vi "Read Voltage.vi"(8 "error in (no error)":errorcluster, 11 "Generic DAQ in":refnum<class "Generic DAQ.lvclass">) -> (0 "error out":errorcluster, 2 "Voltage":dbl, 3 "Generic DAQ out":refnum<class "Generic DAQ.lvclass">)   [LabVIEW 2020, in "Generic DAQ.lvclass"]
uses:
  Generic DAQ.lvclass
  <vilib>/numeric/Random Number (Range) DBL.vi
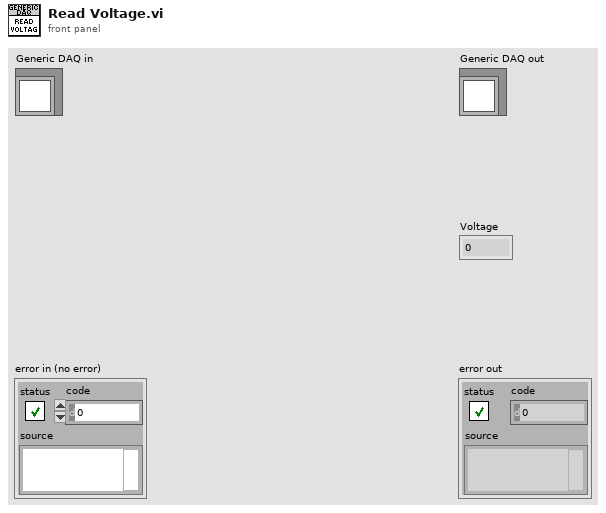
[diagram p1: front panel]
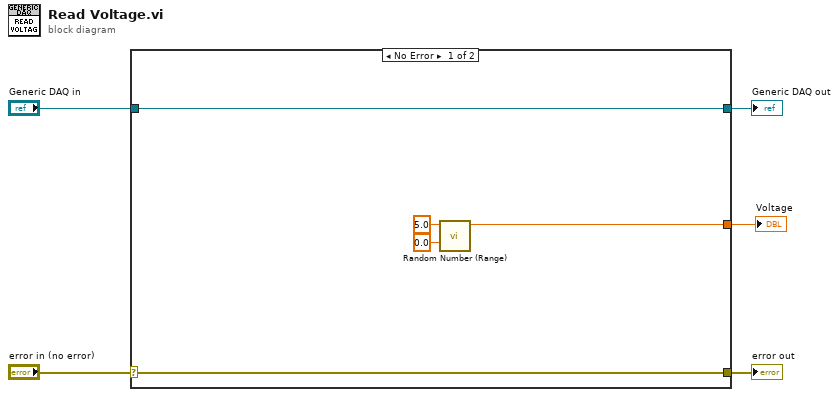
[diagram p0: block diagram]
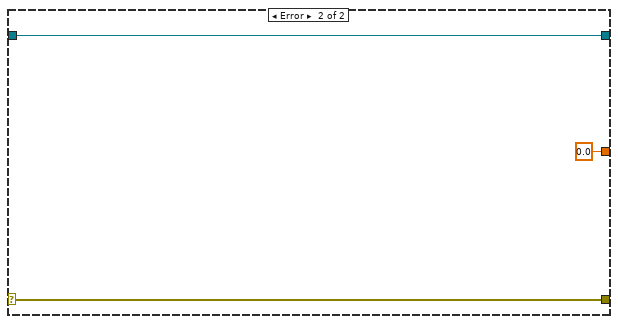
[diagram p2: hidden frame]
diagram:
  n1 = case shown="No Error" "error in (no error)" {
    selector: "error in (no error)" -> [w9 w13]
    tunnel: [w9 w13] -> w4
    tunnel: [w10 w12] -> w2
    tunnel: "Generic DAQ in" -> [w10 w12]
    tunnel: [w6 0.0 ("number")] -> w1
    frame No Error {
      n2 = call-poly <vilib>:"Random Number (Range).vi"("lower bound (0)"=0.0, "upper bound (100)"=5.0) -> ("number"=w6:dbl)  [unwired: 9 in]
    }
    frame Error {
    }
  }
  "error out" <- w4
  "Generic DAQ out" <- w2
  "Voltage" <- w1
